vi "GaGe_TimeoutFill.vi"(10 "TimeOut (s)":sgl, 11 "GaGe Handle":T1) -> (2 "String":string, 3 "GaGe Handle Out":T1)   [LabVIEW 2022 SP3]
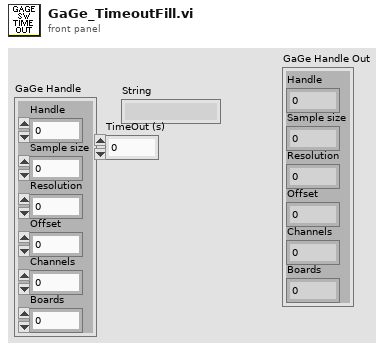
[diagram p1: front panel]
types:
  T1 = cluster{"Handle":u32, "Sample size":u32, "Resolution":i32, "Offset":i32, "Channels":u32, "Boards":u32}
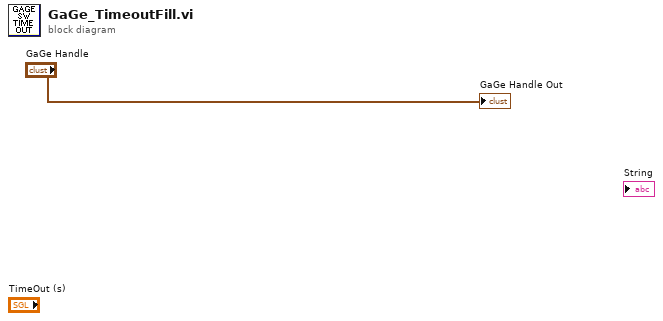
[diagram p0: block diagram]
diagram:
  "GaGe Handle Out" <- "GaGe Handle"
